vi "ChangeDirection.vi"(11 "MainCluster_IN":T11) -> (2 "DirectionChanged":bool, 3 "MainCluster_OUT":T11)   [LabVIEW 2022 SP3]
uses:
  InitCluster.ctl
  CharacterCluster.ctl
  <vilib>/picture/picture.llb/imagedata.ctl
  ShotInitCluster.ctl
  <vilib>/Utility/miscctls.llb/LVPositionTypeDef.ctl
  <vilib>/Utility/miscctls.llb/LVBoundsTypeDef.ctl
  ShotCluster.ctl
  move_dir_ud.ctl
  InvaderPositionArray.ctl
  move_dir_lr.ctl
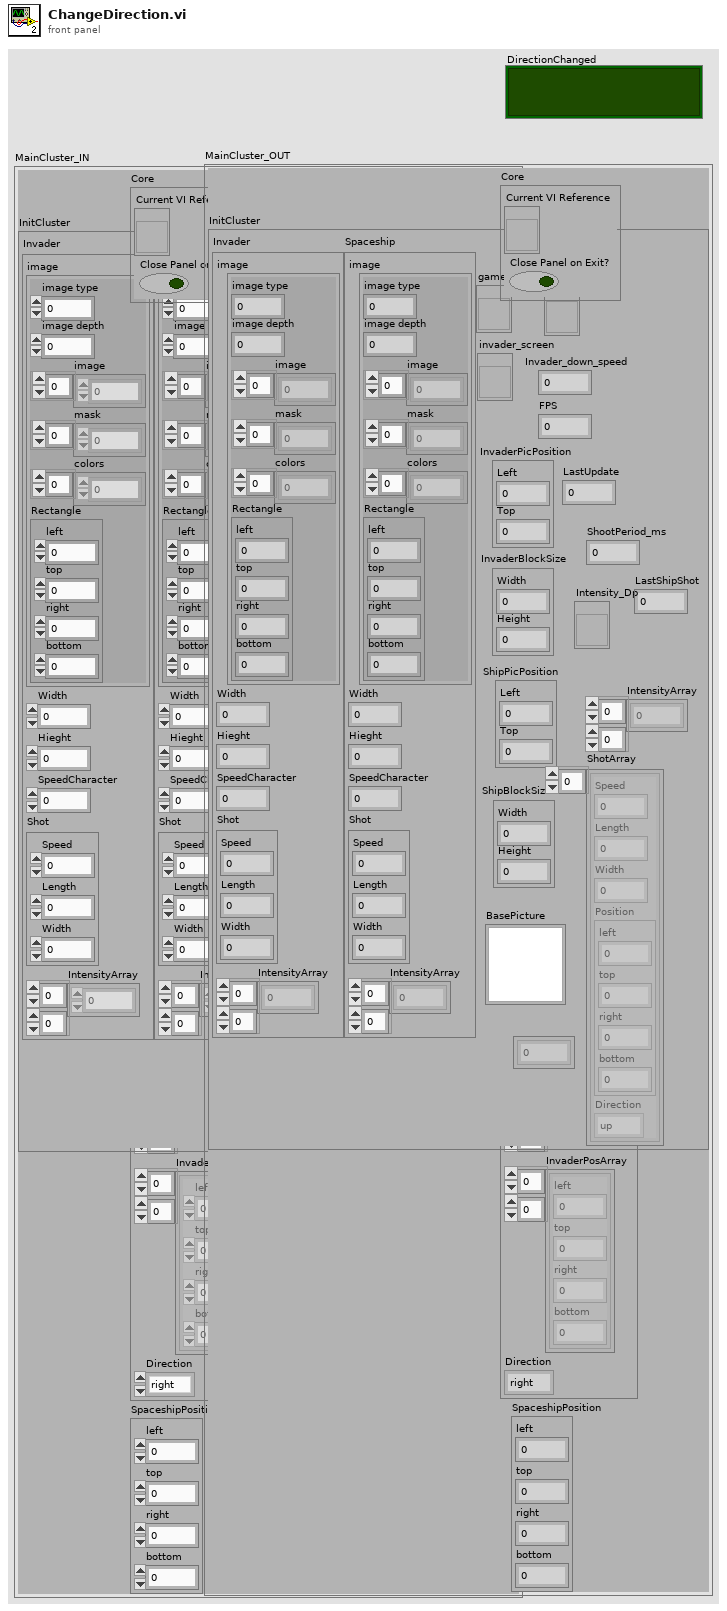
[diagram p1: front panel]
types:
  T1 = typedef "InitCluster.ctl" = cluster{"Invader":T2, "Spaceship":T2, "game_screen":refnum<vi>, "BasePicture":picture, "invader_screen":refnum<vi>, "InvaderPicPosition":T5, "Invader_down_speed":i16, "FPS":u16, "InvaderBlockSize":T6, "ship_screen":refnum<vi>, "ShipBlockSize":T6, "ShipPicPosition":T5, "LastUpdate":u32, "Intensity_Dp":refnum<vi>, "IntensityArray":u8[][], "ShotArray":T7[], "InvaderShotTimeArray":u32[], "ShootPeriod_ms":i32, "LastShipShot":u32}
  T2 = typedef "CharacterCluster.ctl" = cluster{"image":T3, "Width":u32, "Hieght":u32, "SpeedCharacter":u32, "Shot":T4, "IntensityArray":u8[][]}
  T3 = typedef "imagedata.ctl" = cluster{"image type":i32, "image depth":i32, "image":u8[], "mask":u8[], "colors":u32[], "Rectangle":cluster{"left":i16, "top":i16, "right":i16, "bottom":i16}}
  T4 = typedef "ShotInitCluster.ctl" = cluster{"Speed":u32, "Length":u32, "Width":u32}
  T5 = typedef "LVPositionTypeDef.ctl" = cluster{"Left":i32, "Top":i32}
  T6 = typedef "LVBoundsTypeDef.ctl" = cluster{"Width":u32, "Height":u32}
  T7 = typedef "ShotCluster.ctl" = cluster{"Speed":u32, "Length":u32, "Width":u32, "Position":cluster{"left":i16, "top":i16, "right":i16, "bottom":i16}, "Direction":T8}
  T8 = typedef "move_dir_ud.ctl" = enum16{"up", "down"}
  T9 = typedef "InvaderPositionArray.ctl" = cluster{"InvaderAlive":bool[][], "InvaderPosArray":cluster{"left":i16, "top":i16, "right":i16, "bottom":i16}[][], "Direction":T10}
  T10 = typedef "move_dir_lr.ctl" = enum16{"right", "left"}
  T11 = cluster{"Core":cluster{"Current VI Reference":refnum<vi>, "Close Panel on Exit?":bool}, "InitCluster":T1, "InvaderPosArray":T9, "SpaceshipPosition":cluster{"left":i16, "top":i16, "right":i16, "bottom":i16}}
  T12 = cluster{"left":i16, "top":i16, "right":i16, "bottom":i16}
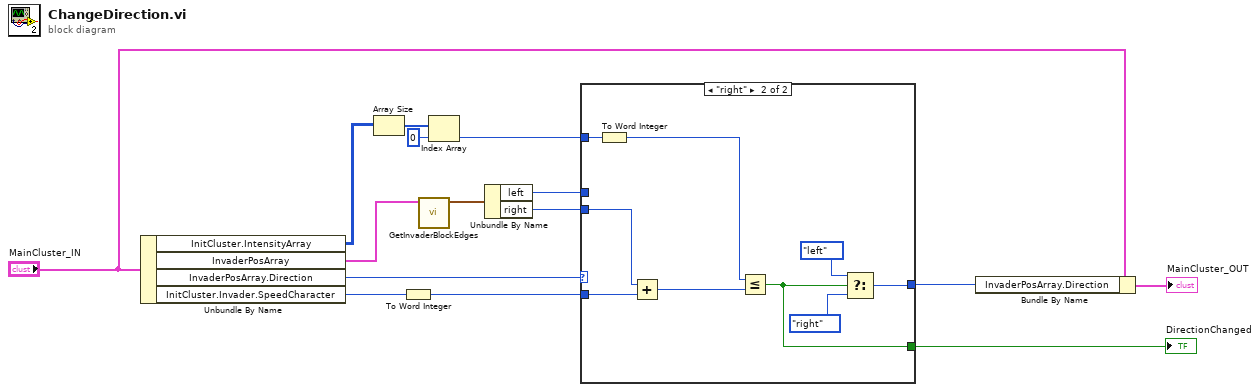
[diagram p0: block diagram]
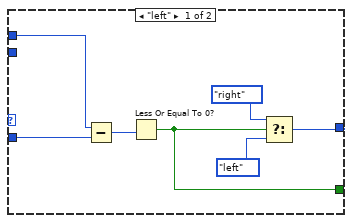
[diagram p2: hidden frame]
diagram:
  n1 = Unbundle By Name("MainCluster_IN") -> ("InitCluster.IntensityArray"=w4:u8[][], "InvaderPosArray"=w15:T9, "InvaderPosArray.Direction"=w13:T10, "InitCluster.Invader.SpeedCharacter"=w11:u32)
  n2 = Array Size(array=w4) -> (size(s)=w3:i32[])
  n3 = To Word Integer(number=w11) -> (16bit integer=w10:i16)
  n4 = call "GetInvaderBlockEdges.vi"("InvaderPosArray"=w15) -> ("output cluster"=w14:T12)  [unwired: 10 in]
  n5 = Index Array(array=w3, index=0) -> (element=w1:i32)
  n6 = Unbundle By Name(w14) -> ("left"=w12:i16, "right"=w5:i16)
  n7 = case shown="\"right\"" w13 {
    tunnel: w12 -> [w19 _]
    tunnel: w10 -> [w18 w26]
    tunnel: [w20 w29] -> w8
    tunnel: [w16 w28] -> w7
    tunnel: w5 -> [_ w25]
    tunnel: w1 -> [_ w27]
    frame "left" {
      n8 = Subtract(x=w19, y=w18) -> (x-y=w17:i16)
      n9 = Less Or Equal To 0?(x=w17) -> (x <= 0?=w16:bool)
      n10 = Select(t=move_dir_lr."right" ("InvaderPosArray.Direction"), s=w16, f=move_dir_lr."left") -> (s? t:f=w20:T10)
    }
    frame "right" {
      n11 = To Word Integer(number=w27) -> (16bit integer=w23:i16)
      n12 = Add(x=w25, y=w26) -> (x+y=w24:i16)
      n13 = Less Or Equal?(x=w23, y=w24) -> (x <= y?=w28:bool)
      n14 = Select(t=move_dir_lr."left" ("InvaderPosArray.Direction"), s=w28, f=move_dir_lr."right") -> (s? t:f=w29:T10)
    }
  }
  "DirectionChanged" <- w7
  n15 = Bundle By Name(cluster="MainCluster_IN", "InvaderPosArray.Direction"=w8) -> (→"MainCluster_OUT":T11)
